vi "FRF.vi"(0 "System no.":i32=1 min=1 max=4 step=1, 2 "Affected axes":string[](array[string]), 3 "All axes?":bool, 4 "Axis identifier?":bool=TRUE, 5 "error in":errorcluster) -> (19 "error out":errorcluster)   [LabVIEW 2020]
doc: "GCS 3.0\n=====\n\nFRF (Start Reference Motion) \n\nDescription\nActivates/deactivates the axis by switching its drive on/off.\nMotion of the axis is only possible if the axis is activated with EAX. Activating with EAX \npasses the axis from the Ready to switch state to the Operation enabled state. For further \ndetails, see \"Drive State Machine\". \n\nFormat\nFRF[ <AxisID>]\n\nArguments\nFRF without arguments starts a reference move for all axes of the controller. The axes start \nsimultaneously.\n<AxisID>\nAn axis of the controller\nThe response to USG? CMD FRF indicates in the #Related Units block for which axes the \ncommand can be used.\nPossible values: Alias of the axis\n\nResponse\nnone\n\nExample\n>>FRF?\n<<AXIS_1=0\n<<AXIS_2=0\n>>FRF\n>>FRF?\n<<AXIS_1=0 \n<<AXIS_2=0\n>>STV?\n<<AXIS_1=0x0\n<<AXIS_2=0x0\n<<SYS_1=0x1\n>>ERR?\n<<49173 - (error 49173 - \"Axis is disabled\")\n>>EAX Axis_1 1\n>>EAX Axis_2 1\n>>FRF?\n<<AXIS_1=0\n<<AXIS_2=0\n>>STV?\n<<AXIS_1=0x2\n<<AXIS_2=0x2\n<<SYS_1=0x0\n>>FRF\n>>STV?\n<<AXIS_1=0x4402A\n<<AXIS_2=0x4402A\n<<SYS_1=0x0\n>>STV?\n<<AXIS_1=0x1002\n<<AXIS_2=0x1002\n<<SYS_1=0x0\n>>FRF?\n<<AXIS_1=1\n<<AXIS_2=1\n\nNotes\nThe reference move is only executed if the following conditions are fulfilled for the specified \naxis (for all axes if no axis is specified):\n- The axis is in the Operation enabled state.\n- The mode of operation is set to Open (0x0).\nFor further details, see \"Drive State Machine\". \nYou can query whether an axis is referenced using the FRF? command. This information \nis also displayed in bit 12 \"FRF?\" of the status register of the axis, which can be queried\nwith the STV? command. \nThe FRF command starts a process and thus sets bit 14 \"IPR\" of the status register of the axis.\nThe reference move can be stopped with the STP and HLT commands.\n\nUser command level\nUSR\n\n\nGCS 2.0\n=====\n\nThis VI starts a fast referencing of the specified axes. Use #7 polling to determine end of this referencing procedure.\n\nC-843, C-843.PM, C-880: If All axes? = TRUE, then Axis identifier? must be TRUE\n\nC-880K005: VI only supported when called through PI_Multix.vi\n\nC-413, C-867, C-877, C-884, E-871, E-873, E-874, Hydra, Pollux, Mercury_GCS: If All axes? = TRUE, then Axis identifier? must be TRUE. Servo must be enabled with SVO for the commanded axis prior to using this command (closed-loop operation).\nThe reference mode must be set to \"1\" (factory default) with the RON command if referencing is to be done by performing a reference move. \nThe value of the VALUE_AT_REF_POS parameter (ID 0x16) is set as the current position when the axis is at the reference switch. Use FNL or FPL (if supported) instead of FRF to perform a reference move for an axis which has no reference sensor but limit switches. See user manual for details and specifics. \n\nC-885: If All axes? = TRUE, then Axis identifier? can be FALSE. Servo must be enabled with SVO for the commanded axis prior to using this command (closed-loop operation).\nThe reference mode must be set to \"1\" (factory default) with the RON command if referencing is to be done by performing a reference move. \n\nC-886: If All axes? = TRUE, then Axis identifier? can be FALSE. Servo must be enabled with SVO for additional axes prior to using this command (closed-loop operation).\n\nC-891: If All axes? = TRUE, then Axis identifier? must be TRUE. The system mechanics Reference type can be set by changing the parameter ID 0x70. For details please refer to the Controller user manual.\n\nE-712: If All axes? = TRUE, then Axis identifier? must be TRUE. \n\nE-861: If All axes? = TRUE, then Axis identifier? must be TRUE. The reference mode must be set to \"1\" (factory default) with the RON command if referencing is to be done by performing a reference move. \nThe value of the VALUE_AT_REF_POS parameter (ID 0x16) is set as the current position when the axis is at the reference switch. Use FNL or FPL (if supported) instead of FRF to perform a reference move for an axis which has no reference sensor but limit switches.\n\nC-887, F-206, M-8X0: If All axes? = TRUE, then Axis identifier? must be TRUE. Only for GCS syntax version = GCS 2.0 or higher (check with CSV?.vi. If CSV?.vi is not supported, syntax version is GCS 1.0). For GCS syntax version = GCS 1.0 use INI.vi for initialization."
panel:
  # "FRF (Start Reference Motion)\n\nActivates/deactivates the axis by switching its drive on/off.\nMotion of the axis is only possible if the axis is activated with EAX.\nActivating with EAX passes the axis from the Ready to switch state to the\nOperation enabled state. For further details, see \"Drive State Machine\"."
  # "If all axes: use"
  # "FRF"
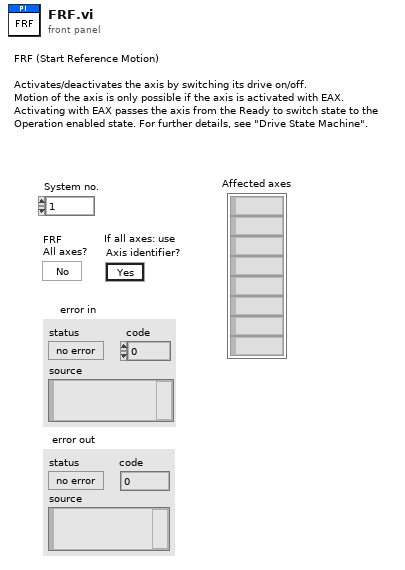
[diagram p1: front panel]
types:
  T1 = typedef "Syntax.ctl" = enum16{"GCS 1.0", "GCS 2.0", "GCS 3.0"}
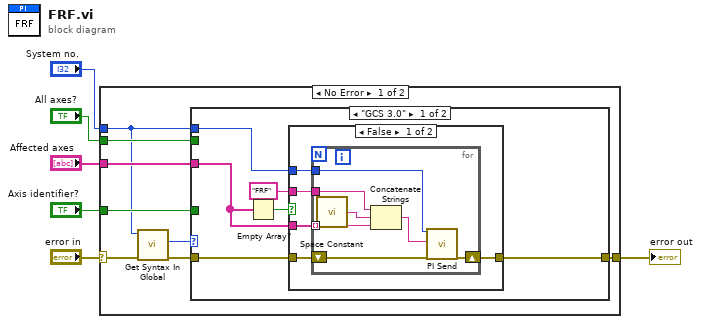
[diagram p0: block diagram]
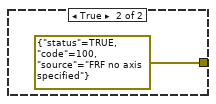
[diagram p2: hidden frame]
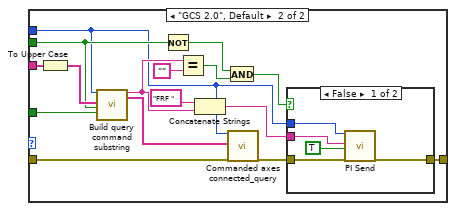
[diagram p3: hidden frame]
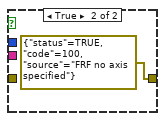
[diagram p4: hidden frame]
diagram:
  n1 = case shown="No Error" "error in" {
    selector: "error in" -> [w10 w56]
    tunnel: "Affected axes" -> [w14 _]
    tunnel: [w13 w56] -> w5
    tunnel: "Axis identifier?" -> [w12 _]
    tunnel: "System no." -> [w8 _]
    tunnel: "All axes?" -> [w11 _]
    frame No Error {
      n2 = call "Get Syntax In Global.vi"("error in"=w10, "System no."=w8) -> ("error out"=w9:errorcluster, "Syntax"=w7:T1)  [unwired: 8 in]
      n3 = case shown="\"GCS 3.0\"" w7 {
        tunnel: w14 -> [w16 w48]
        tunnel: [w20 w45] -> w13
        tunnel: w12 -> [_ w43]
        tunnel: w11 -> [_ w40]
        tunnel: w9 -> [w19 w35]
        tunnel: w8 -> [w18 w34]
        frame "GCS 3.0" {
          n4 = Empty Array?(array=w16) -> (empty?=w15:bool)
          n5 = case shown="False" w15 {
            tunnel: [w25 errorcluster {"status"=TRUE, "code"=100, "source"="FRF no axis specified"} ("error out")] -> w20
            tunnel: w19 -> [w24 _]
            tunnel: w16 -> [w23 _]
            tunnel: w18 -> [w22 _]
            tunnel: "FRF" -> [w21 _]
            frame False {
              n6 = for {
                shift-right: [w32] -> w25
                shift-left: w24 -> [w31]
                tunnel: w23 -> [w28] mode=indexing
                tunnel: w22 -> [w30]
                tunnel: w21 -> [w27]
                n7 = call "Space Constant.vi"() -> ("String"=w29:string)
                n8 = Concatenate Strings(w27, w29, w28) -> (w26:string)
                n9 = call "PI Send.vi"("System no."=w30, "String to send"=w26, "error in"=w31) -> ("error out"=w32:errorcluster)  [unwired: 3 in, 13 out]
              }
            }
            frame True {
            }
          }
        }
        frame "GCS 2.0", Default {
          n10 = To Upper Case(1:w48) -> (0:w44:string[])
          n11 = call "Build query command substring.vi"("System no."=w34, "Axes to query in"=w44, "Query\nAll axes?"=w40, "For all axes: use\nAxis identifier?"=w43) -> ("Command substring"=w42:string, "Axes to query out"=w41:string[])  [unwired: 2 in, 12 out]
          n12 = Not(x=w40) -> (.not. x?=w38:bool)
          n13 = Equal?(x=w42, y="" ("x")) -> (x = y?=w39:bool)
          n14 = Concatenate Strings("FRF ", w42) -> (w36:string)
          n15 = And(x=w38, y=w39) -> (x .and. y?=w46:bool)
          n16 = call "Commanded axes connected_query.vi"("System no."=w34, "Commanded axes"=w41, "error in"=w35) -> ("error out"=w37:errorcluster)  [unwired: 1 in, 15 out]
          n17 = case shown="False" w46 {
            tunnel: [w50 errorcluster {"status"=TRUE, "code"=100, "source"="FRF no axis specified"} ("error out")] -> w45
            tunnel: w37 -> [w54 _]
            tunnel: w36 -> [w52 _]
            tunnel: w34 -> [w51 _]
            frame False {
              n18 = call "PI Send.vi"("System no."=w51, "String to send"=w52, "Attach termination char.?"=TRUE ("Attach Linefeed?"), "error in"=w54) -> ("error out"=w50:errorcluster)  [unwired: 2 in, 13 out]
            }
            frame True {
            }
          }
        }
      }
    }
    frame Error {
    }
  }
  "error out" <- w5
